vi "Exercice4Operations.vi"() -> ()   [LabVIEW 2018]
panel:
  out "a / b":dbl(knob) scale=0.0..9.0
  out "a * b":i8(slide) scale=0.0..81.0
  out "a-b":i8(knob) scale=-9.0..9.0
  out "a+b":i8
  in  "b":i8(slide) scale=0.0..9.0
  in  "a":i8 min=0 max=9
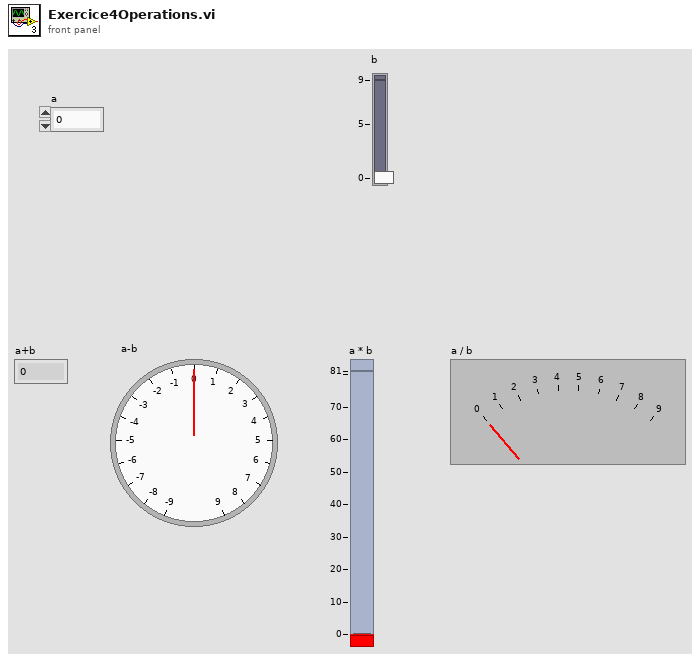
[diagram p1: front panel]
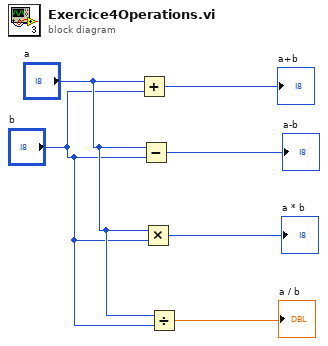
[diagram p0: block diagram]
diagram:
  n1 = Add(x="a", y="b") -> (x+y=→"a+b":i8)
  n2 = Subtract(x="a", y="b") -> (x-y=→"a-b":i8)
  n3 = Multiply(x="a", y="b") -> (x*y=→"a * b":i8)
  n4 = Divide(x="a", y="b") -> (x/y=→"a / b":dbl)
